vi "Layer_Set Active Data BG Color.vi"(7 "Highlight Color":T1, 8 "error in":errorcluster, 9 "Highlighted Indices":u32[](array[numeric]), 11 "Cluster Refnum":refnum<vi>) -> (0 "error out":errorcluster)   [LabVIEW 2021, in "FakedArray.lvclass"]
uses:
  <resource>/plugins/NIIconEditor/Class/FakedArray/FakedArray.lvclass
  <vilib>/LabVIEW Icon API/lv_icon/Controls/IEColor.ctl
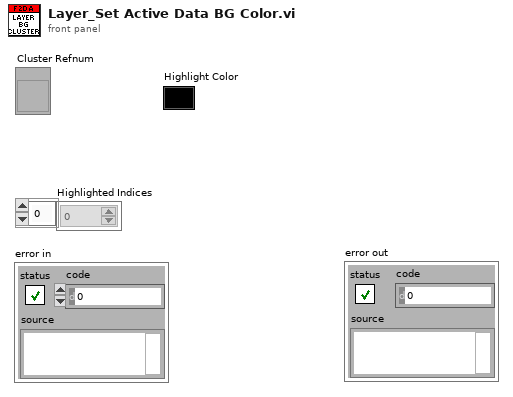
[diagram p1: front panel]
types:
  T1 = typedef "IEColor.ctl" = u32
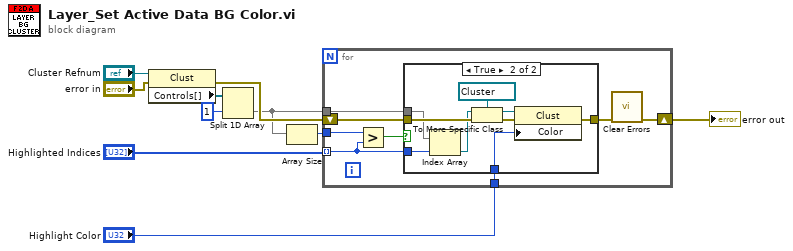
[diagram p0: block diagram]
diagram:
  n1 = property class="Clust"(reference="Cluster Refnum", error in="error in") -> (error out=w4:errorcluster, "Controls[]"=w5:refnum<vi>[])  [unwired: 1 out]
  n2 = Split 1D Array(array=w5, index=1) -> (second subarray=w2:refnum<vi>[])  [unwired: 1 out]
  n3 = Array Size(array=w2) -> (size(s)=w1:i32)
  n4 = for {
    shift-right: [w14] -> w9
    shift-left: w4 -> [w18]
    tunnel: "Highlighted Indices" -> [w12] mode=indexing
    tunnel: w2 -> [w17]
    tunnel: "Highlight Color" -> [w16]
    tunnel: w1 -> [w13]
    n5 = Greater?(x=w13, y=w12) -> (0:w11:bool)
    n6 = case shown="True" w11 {
      tunnel: w18 -> [w19 w28]
      tunnel: w17 -> [_ w27]
      tunnel: w16 -> [_ w26]
      tunnel: [w19 w25] -> w15
      tunnel: w12 -> [_ w20]
      frame False {
      }
      frame True {
        n7 = Index Array(array=w27, index=w20) -> (element=w21:refnum<vi>)
        n8 = To More Specific Class(target class=refnum<vi> refnum ("Clust Refnum"), reference=w21, error in=w28) -> (specific class reference=w23:refnum<vi>, error out=w22:errorcluster)
        n9 = property class="Clust"(reference=w23, error in=w22, "Color"=w26) -> (error out=w25:errorcluster)  [unwired: 1 out]
      }
    }
    n10 = call <vilib>:"Clear Errors.vi"("error in (no error)"=w15) -> ("error out"=w14:errorcluster)  [unwired: 1 in, 5 out]
  }
  "error out" <- w9
